vi "Main.vi"() -> ()   [LabVIEW 2018]
uses:
  Ddigit--enum.ctl
  Mmultiplier--enum.ctl
  Ttolerance--enum.ctl
  Number of Bands--number.ctl
  Ttemp Ccoeficient--enum.ctl
  In series--cluster.ctl
  Data--cluster.ctl
  E-Series Reader/Series Data--cluster.ctl
  Resistance Digits--cluster.ctl
  <vilib>/TABOADA/Event-Driven Queued SM/ED Queued State Machine/Queue State & Data (Array).vi
  <vilib>/Utility/error.llb/Error Cluster From Error Code.vi
  <vilib>/TABOADA/Event-Driven Queued SM/ED Queued State Machine/Queue State & Data (Single).vi
  <vilib>/ErrorRing/Error Ring.xnode
  Enum to Color Converters/Enum to Color Converters.lvlib
  E-Series Reader/E-Series Reader.lvlib
  Resistance Value/Resistance Value.lvlib
  Front Panel Interface/Front Panel Interface.lvlib
  <vilib>/TABOADA/Event-Driven Queued SM/ED Queued State Machine/ED Queued State Machine.lvlib
panel:
  out "RNV":dbl format="%#_6p"
  in  "Exit":bool
  out "T Rge":dbl caption="Tol Range [Ohm]" format="%_2p"
  out "Dev":dbl caption="Deviation [Ohm]" format="%_2p"
  out "UL":dbl caption="Upper Limit [Ohm]" format="%_3p"
  out "LL":dbl caption="Lower Limit [Ohm]" format="%_3p"
  out "Tol %":dbl caption="Tolerance (%)"
  out "In S":T1 caption="In Series"
  in  "Series Data File Name":string="e-series files names.ini"
  out "TC col":u32(colorbox) caption="TC"
  out "3D col":u32(colorbox) caption="3D"
  out "Tol col":u32(colorbox) caption="Tol"
  out "M col":u32(colorbox) caption="M"
  out "2D col":u32(colorbox) caption="2D"
  out "1D col":u32(colorbox) caption="1D"
  in  "Temp Coef":T2
  in  "3° Digit":T3
  in  "# Bands":T4=3 caption="Number of Bands" min=3 max=6 step=1
  out "N Val":dbl caption="Nominal [Ohm]" format="%#_3p"
  in  "Tolerance":T5=enum."Gold - 5%"
  in  "Multiplier":T6
  in  "2° Digit":T3
  in  "1° Digit":T3
  # "Resistor graphical representation"
  # "User Data Input"
  # "Calculated Resistor Specifications"
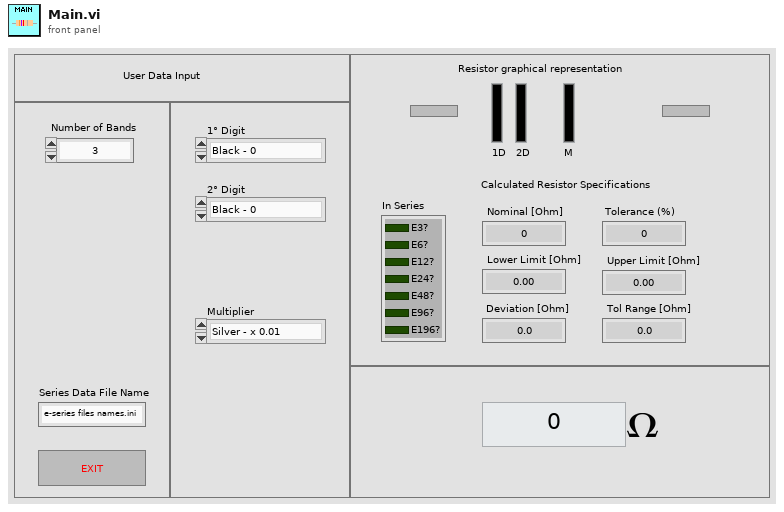
[diagram p1: front panel]
types:
  T1 = typedef "In series--cluster.ctl" = cluster{"E3?":bool, "E6?":bool, "E12?":bool, "E24?":bool, "E48?":bool, "E96?":bool, "E196?":bool}
  T2 = typedef "Ttemp Ccoeficient--enum.ctl" = enum16{"Grey - 1 ppm/K", "Violet - 5 ppm/K", "Blue - 10 ppm/K", "Green - 20 ppm/K", "Yellow - 25 ppm/K", "Orange - 15 ppm/K", "Red - 50 ppm/K", "Brown - 100 ppm/K", "Black - 250 ppm/K"}
  T3 = typedef "Ddigit--enum.ctl" = enum16{"Black - 0", "Brown - 1", "Red - 2", "Orange - 3", "Yellow - 4", "Green - 5", "Blue - 6", "Violet - 7", "Grey - 8", "White - 9"}
  T4 = typedef "Number of Bands--number.ctl" = u8
  T5 = typedef "Ttolerance--enum.ctl" = enum16{"Gray - 0.05%", "Violet - 0.1%", "Blue - 0.25%", "Green - 0.5%", "Brown - 1%", "Red - 2%", "Gold - 5%", "Silver - 10%", "None - 20%"}
  T6 = typedef "Mmultiplier--enum.ctl" = enum16{"Silver - x 0.01", "Gold - x 0.1 ", "Black - x 1", "Brown - x 10", "Red - x 100", "Orange - x 1k", "Yellow - x 10k", "Green - 100k", "Blue - x 1M", "Violet - x10 M", "Grey - x 100M", "White - x 1G"}
  T7 = typedef "Data--cluster.ctl" = cluster{"1D sel Refn":refnum<vi>, "2D sel Refn":refnum<vi>, "3D sel Refn":refnum<vi>, "M sel Refn":refnum<vi>, "Tol sel Refn":refnum<vi>, "TC sel Refn":refnum<vi>, "# Bands Refn":refnum<vi>, "1D col Refn":refnum<vi>, "2D col Refn":refnum<vi>, "3D col Refn":refnum<vi>, "M col Refn":refnum<vi>, "Tol col Refn":refnum<vi>, "TC col Refn":refnum<vi>, "# Bands":T4, "E-Series Data":T8, "In Series?":T1, "1D sel":T3, "2D sel":T3, "3D sel":T3, "M sel":T6, "Tol sel":T5, "TC sel":T2, "Tol %":dbl, "1D col":u32, "2D col":u32, "3D col":u32, "M col":u32, "Tol col":u32, "TC col":u32, "Nom Value":dbl, "Up Limit":dbl, "Lo Limit":dbl, "Deviation":dbl, "Tol Rge":dbl}
  T8 = typedef "E-Series Reader.lvlib/Series Data--cluster.ctl" = cluster{"E3":u16[], "E6":u16[], "E12":u16[], "E24":u16[], "E48":u16[], "E96":u16[], "E192":u16[]}
  T9 = typedef "Resistance Digits--cluster.ctl" = cluster{"LSD Digit":T3, "MID Digit":T3, "MSD Digit":T3}
  T10 = typedef "digit--enum.ctl" = enum16{"Black - 0", "Brown - 1", "Red - 2", "Orange - 3", "Yellow - 4", "Green - 5", "Blue - 6", "Violet - 7", "Grey - 8", "White - 9"}
  T11 = typedef "multiplier--enum.ctl" = enum16{"Silver - x 0.01", "Gold - x 0.1 ", "Black - x 1", "Brown - x 10", "Red - x 100", "Orange - x 1k", "Yellow - x 10k", "Green - 100k", "Blue - x 1M", "Violet - x10 M", "Grey - x 100M", "White - x 1G"}
  T12 = typedef "tolerance--enum.ctl" = enum16{"Gray - 0.05%", "Violet - 0.1%", "Blue - 0.25%", "Green - 0.5%", "Brown - 1%", "Red - 2%", "Gold - 5%", "Silver - 10%", "None - 20%"}
  T13 = typedef "temp coeficient--enum.ctl" = enum16{"Grey - 1 ppm/K", "Violet - 5 ppm/K", "Blue - 10 ppm/K", "Green - 20 ppm/K", "Yellow - 25 ppm/K", "Orange - 15 ppm/K", "Red - 50 ppm/K", "Brown - 100 ppm/K", "Black - 250 ppm/K"}
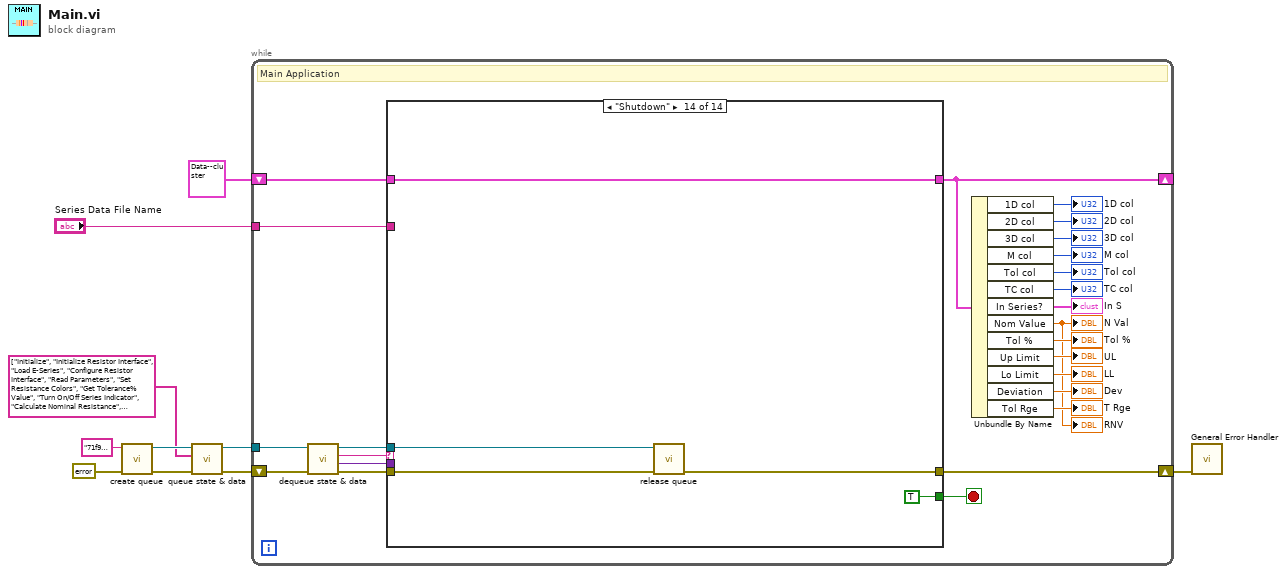
[diagram p0: block diagram]
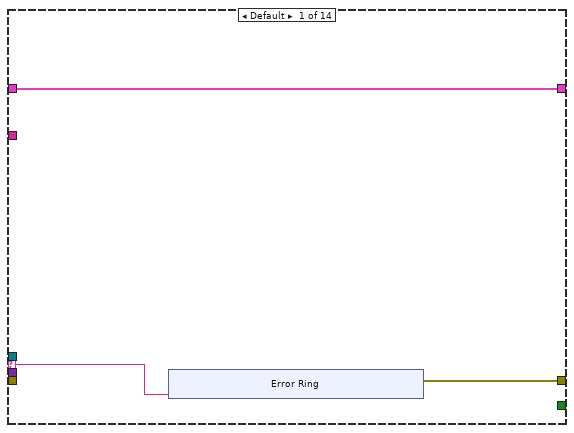
[diagram p2: hidden frame]
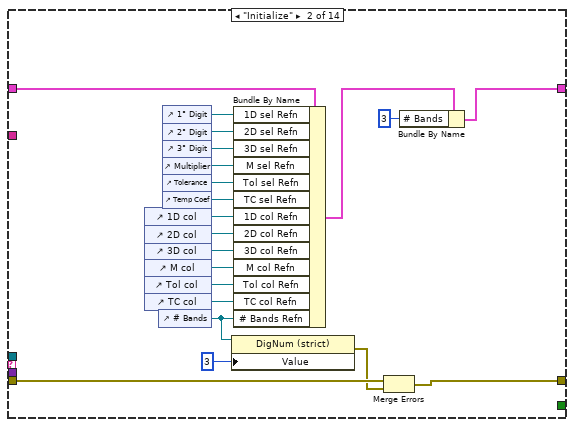
[diagram p3: hidden frame]
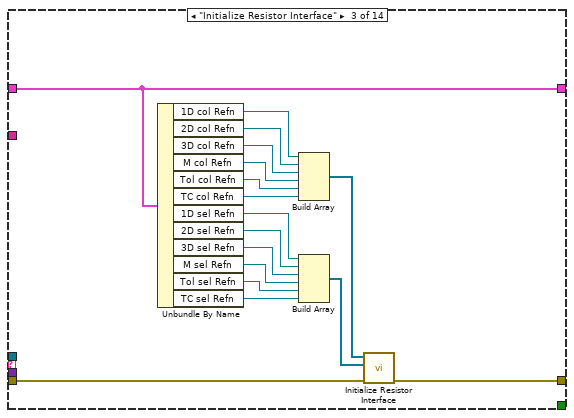
[diagram p4: hidden frame]
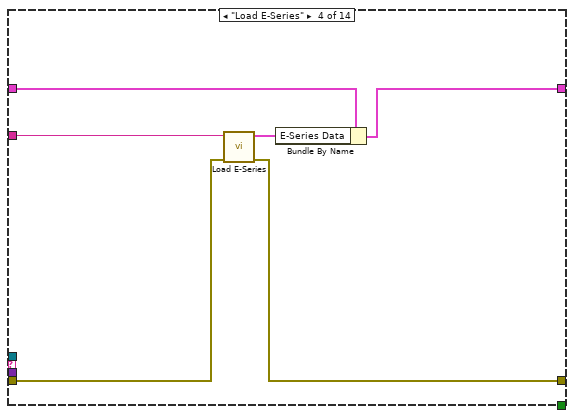
[diagram p5: hidden frame]
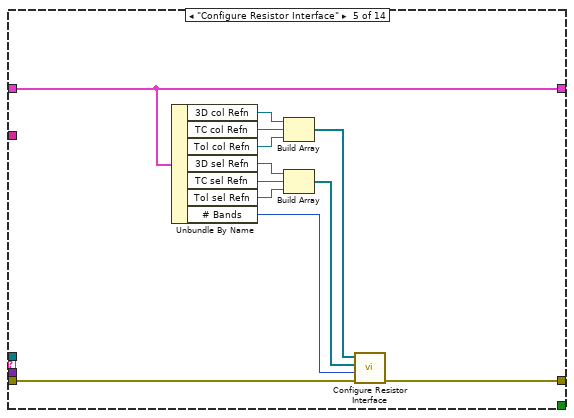
[diagram p6: hidden frame]
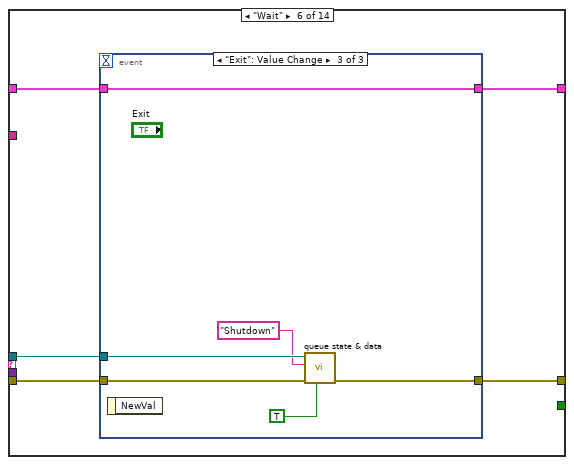
[diagram p7: hidden frame]
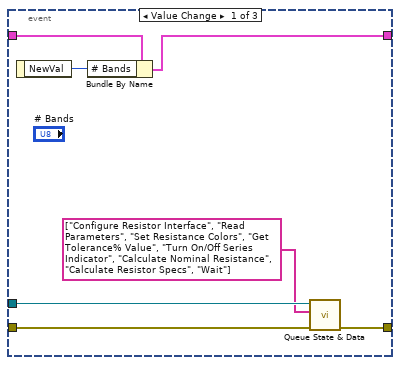
[diagram p8: hidden frame]
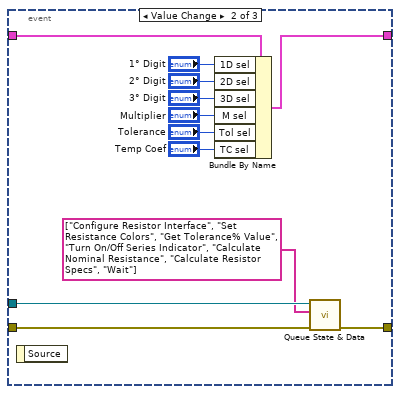
[diagram p9: hidden frame]
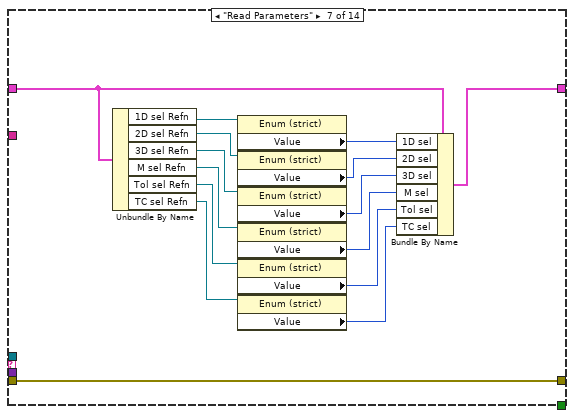
[diagram p10: hidden frame]
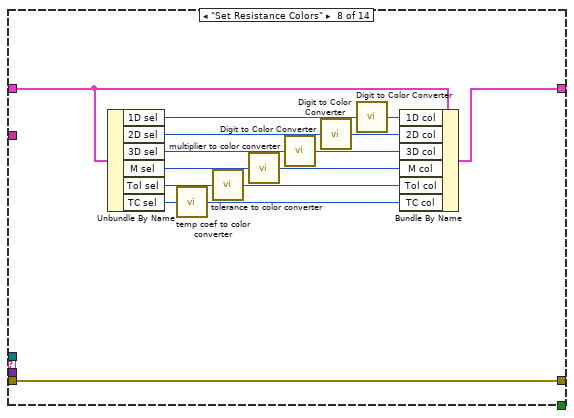
[diagram p11: hidden frame]
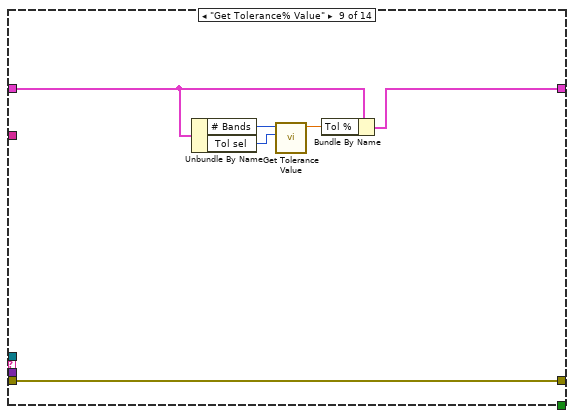
[diagram p12: hidden frame]
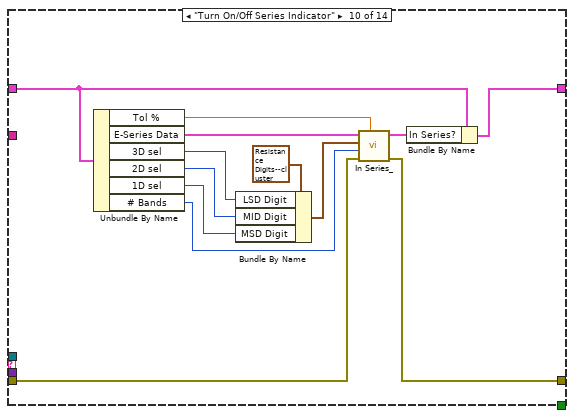
[diagram p13: hidden frame]
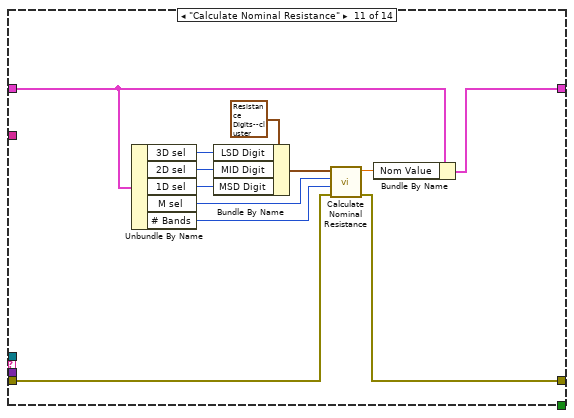
[diagram p14: hidden frame]
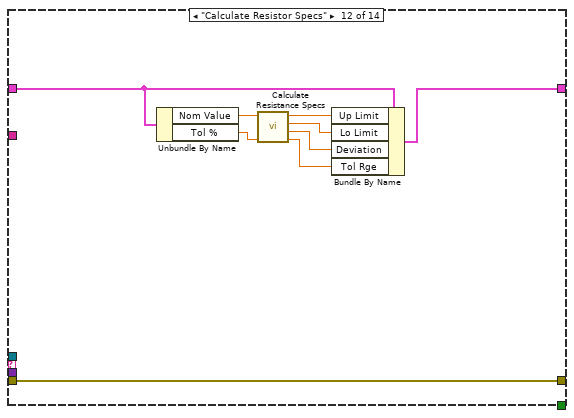
[diagram p15: hidden frame]
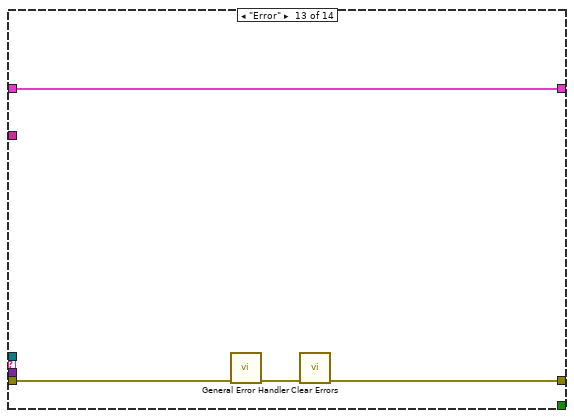
[diagram p16: hidden frame]
diagram:
  n1 = call <vilib>:"create queue.vi"("error in (no error)"=errorcluster {"status"=FALSE, "code"=0, "source"=""} ("error constant"), "name (unnamed)"="71f9ea68-780e-483a-a5bb-45874721e19e") -> ("error out"=w6:errorcluster, "queue out"=w4:refnum<queue>)  [unwired: 7 in, 1 out]
  n2 = call-poly <vilib>:"queue state & data.vi"("error in (no error)"=w6, "State Array"=string[] ["Initialize", "Initialize Resistor Interface", "Load E-Series", "Configure Resistor Interface", "Read Parameters", "Set Resistance Colors", "Get Tolerance% Value", "Turn On/Off Series Indicator", "Calculate Nominal Resistance", "Calculate Resistor Specs", "Wait"], "queue in"=w4) -> ("error out"=w7:errorcluster, "queue out"=w3:refnum<queue>)  [unwired: 7 in]
  n3 = while {
    shift-right: [w34] -> w9
    shift-left: w7 -> [w22]
    shift-right: [w24] -> _
    shift-left: T7 {"1D sel Refn"=refnum, "2D sel Refn"=refnum, "3D sel Refn"=refnum, "M sel Refn"=refnum, "Tol sel Refn"=refnum, "TC sel Refn"=refnum, "# Bands Refn"=refnum, "1D col Refn"=refnum, "2D col Refn"=refnum, "3D col Refn"=refnum, "M col Refn"=refnum, "Tol col Refn"=refnum, "TC col Refn"=refnum, "# Bands"=0, "E-Series Data"={"E3"=[], "E6"=[], "E12"=[], "E24"=[], "E48"=[], "E96"=[], "E192"=[]}, "In Series?"={"E3?"=FALSE, "E6?"=FALSE, "E12?"=FALSE, "E24?"=FALSE, "E48?"=FALSE, "E96?"=FALSE, "E196?"=FALSE}, "1D sel"=enum."Black - 0", "2D sel"=enum."Black - 0", "3D sel"=enum."Black - 0", "M sel"=enum."Silver - x 0.01", "Tol sel"=enum."Gray - 0.05%", "TC sel"=enum."Grey - 1 ppm/K", "Tol %"=0.0, "1D col"=0, "2D col"=0, "3D col"=0, "M col"=0, "Tol col"=0, "TC col"=0, "Nom Value"=0.0, "Up Limit"=0.0, "Lo Limit"=0.0, "Deviation"=0.0, "Tol Rge"=0.0} -> [w25]
    tunnel: "Series Data File Name" -> [w26]
    tunnel: w3 -> [w23]
    stop <- w33 stop-if-true
    # "Main Application"
    n4 = call <vilib>:"dequeue state & data.vi"("error in (no error)"=w22, "queue in"=w23) -> ("error out"=w20:errorcluster, "State Data"=w18:variant, "State"=w19:string, "queue out"=w21:refnum<queue>)  [unwired: 6 in]
    n5 = case shown="\"Shutdown\"" w19 {
      selector: w19 -> [w36 _ _ _ _ _ _ _ _ _ _ _ _ _]
      tunnel: w20 -> [_ w65 w76 w84 w95 w103 w145 w159 w166 w169 w182 w200 w202 w207]
      tunnel: [w35 w49 w75 w86 w96 w102 w145 w159 w166 w168 w181 w200 w203 w206] -> w34
      tunnel: w25 -> [w37 w64 w82 w88 w100 w105 w143 w157 w165 w172 w191 w199 w204 w209]
      tunnel: [w37 w46 w82 w87 w100 w104 w144 w156 w163 w170 w190 w198 w204 w209] -> w24
      tunnel: [_ _ _ _ _ _ _ _ _ _ _ _ _ TRUE] -> w33
      tunnel: w26 -> [_ _ _ w83 _ _ _ _ _ _ _ _ _ _]
      tunnel: w21 -> [_ _ _ _ _ w101 _ _ _ _ _ _ _ w205]
      tunnel: w18 -> [_ _ _ _ _ _ _ _ _ _ _ _ _ _]
      frame Default {
        n6 = xnode ("Error Ring")("parameter 0"=w36) -> ("error out"=w35:errorcluster)
      }
      frame "Initialize" {
        n7 = control-ref of="1D col"() -> (w60:refnum<vi>)
        n8 = control-ref of="2D col"() -> (w59:refnum<vi>)
        n9 = control-ref of="3D col"() -> (w58:refnum<vi>)
        n10 = control-ref of="M col"() -> (w57:refnum<vi>)
        n11 = control-ref of="Tol col"() -> (w56:refnum<vi>)
        n12 = control-ref of="TC col"() -> (w55:refnum<vi>)
        n13 = control-ref of="# Bands"() -> (w51:refnum<vi>)
        n14 = control-ref of="1° Digit"() -> (w52:refnum<vi>)
        n15 = control-ref of="2° Digit"() -> (w53:refnum<vi>)
        n16 = control-ref of="3° Digit"() -> (w54:refnum<vi>)
        n17 = control-ref of="Multiplier"() -> (w63:refnum<vi>)
        n18 = control-ref of="Tolerance"() -> (w62:refnum<vi>)
        n19 = control-ref of="Temp Coef"() -> (w61:refnum<vi>)
        n20 = property class="DigNum (strict)"(reference=w51, "Value"=T4 3 ("Number of Bands")) -> (error out=w48:errorcluster)  [unwired: 1 in, 1 out]
        n21 = Bundle By Name(cluster=w64, "1D sel Refn"=w52, "2D sel Refn"=w53, "3D sel Refn"=w54, "M sel Refn"=w63, "Tol sel Refn"=w62, "TC sel Refn"=w61, "1D col Refn"=w60, "2D col Refn"=w59, "3D col Refn"=w58, "M col Refn"=w57, "Tol col Refn"=w56, "TC col Refn"=w55, "# Bands Refn"=w51) -> (w47:T7)
        n22 = Merge Errors(w65, w48) -> (w49:errorcluster)
        n23 = Bundle By Name(cluster=w47, "# Bands"=T4 3) -> (w46:T7)
      }
      frame "Initialize Resistor Interface" {
        n24 = Unbundle By Name(w82) -> ("1D col Refn"=w81:refnum<vi>, "2D col Refn"=w80:refnum<vi>, "3D col Refn"=w79:refnum<vi>, "M col Refn"=w73:refnum<vi>, "Tol col Refn"=w74:refnum<vi>, "TC col Refn"=w78:refnum<vi>, "1D sel Refn"=w72:refnum<vi>, "2D sel Refn"=w71:refnum<vi>, "3D sel Refn"=w70:refnum<vi>, "M sel Refn"=w69:refnum<vi>, "Tol sel Refn"=w68:refnum<vi>, "TC sel Refn"=w67:refnum<vi>)
        n25 = Build Array(w81, w80, w79, w73, w74, w78) -> (w77:refnum<vi>[])
        n26 = Build Array(w72, w71, w70, w69, w68, w67) -> (w66:refnum<vi>[])
        n27 = call "Initialize Resistor Interface.vi"("error in (no error)"=w76, "Enum Refnum"=w66, "Color Box Refnum"=w77) -> ("error out"=w75:errorcluster)  [unwired: 8 in]
      }
      frame "Load E-Series" {
        n28 = call "Load E-Series.vi"("error in (no error)"=w84, "INI File"=w83) -> ("error out"=w86:errorcluster, "E-Series Data"=w85:T8)  [unwired: 8 in]
        n29 = Bundle By Name(cluster=w88, "E-Series Data"=w85) -> (w87:T7)
      }
      frame "Configure Resistor Interface" {
        n30 = Unbundle By Name(w100) -> ("3D col Refn"=w98:refnum<vi>, "TC col Refn"=w99:refnum<vi>, "Tol col Refn"=w97:refnum<vi>, "3D sel Refn"=w92:refnum<vi>, "TC sel Refn"=w93:refnum<vi>, "Tol sel Refn"=w91:refnum<vi>, "# Bands"=w89:T4)
        n31 = Build Array(w98, w99, w97) -> (w94:refnum<vi>[])
        n32 = Build Array(w92, w93, w91) -> (w90:refnum<vi>[])
        n33 = call "Configure Resistor Interface.vi"("error in (no error)"=w95, "Number of Bands in"=w89, "Enum Refnum"=w90, "Color Box Refnum"=w94) -> ("error out"=w96:errorcluster)  [unwired: 7 in]
      }
      frame "Wait" {
        n34 = event shown="[2] \"Exit\": Value Change" {
          selector: _ -> [_ _ _]
          dyn-events: _ -> [_ _ _]
          timeout: _ -> [_ _ _]
          tunnel: w105 -> [w112 w124 w130]
          tunnel: [w111 w123 w130] -> w104
          tunnel: w103 -> [w109 w116 w128]
          tunnel: [w108 w115 w127] -> w102
          tunnel: w101 -> [w107 w114 w129]
          event Value Change {
            n35 = event-data() -> ("NewVal"=w110:T4)  [unwired: 1 in]
            n36 = Bundle By Name(cluster=w112, "# Bands"=w110) -> (w111:T7)
            n37 = call-poly <vilib>:"Queue State & Data.vi"("error in (no error)"=w109, "State Array"=string[] ["Configure Resistor Interface", "Read Parameters", "Set Resistance Colors", "Get Tolerance% Value", "Turn On/Off Series Indicator", "Calculate Nominal Resistance", "Calculate Resistor Specs", "Wait"], "queue in"=w107) -> ("error out"=w108:errorcluster)  [unwired: 7 in, 1 out]
          }
          event Value Change {
            n38 = event-data() -> ()  [unwired: 1 in, 1 out]
            n39 = Bundle By Name(cluster=w124, "1D sel"="1° Digit", "2D sel"="2° Digit", "3D sel"="3° Digit", "M sel"="Multiplier", "Tol sel"="Tolerance", "TC sel"="Temp Coef") -> (w123:T7)
            n40 = call-poly <vilib>:"Queue State & Data.vi"("error in (no error)"=w116, "State Array"=string[] ["Configure Resistor Interface", "Set Resistance Colors", "Get Tolerance% Value", "Turn On/Off Series Indicator", "Calculate Nominal Resistance", "Calculate Resistor Specs", "Wait"], "queue in"=w114) -> ("error out"=w115:errorcluster)  [unwired: 7 in, 1 out]
          }
          event "Exit": Value Change {
            n41 = event-data() -> ()  [unwired: 1 in, 1 out]
            n42 = call-poly <vilib>:"queue state & data.vi"("Priority State? (F)"=TRUE, "error in (no error)"=w128, "State"="Shutdown", "queue in"=w129) -> ("error out"=w127:errorcluster)  [unwired: 6 in, 1 out]
          }
        }
      }
      frame "Read Parameters" {
        n43 = Unbundle By Name(w143) -> ("1D sel Refn"=w142:refnum<vi>, "2D sel Refn"=w140:refnum<vi>, "3D sel Refn"=w139:refnum<vi>, "M sel Refn"=w136:refnum<vi>, "Tol sel Refn"=w135:refnum<vi>, "TC sel Refn"=w134:refnum<vi>)
        n44 = property class="Enum (strict)"(reference=w142) -> ("Value"=w141:T10)  [unwired: 1 in, 2 out]
        n45 = property class="Enum (strict)"(reference=w140) -> ("Value"=w138:T10)  [unwired: 1 in, 2 out]
        n46 = property class="Enum (strict)"(reference=w139) -> ("Value"=w137:T10)  [unwired: 1 in, 2 out]
        n47 = property class="Enum (strict)"(reference=w136) -> ("Value"=w133:T11)  [unwired: 1 in, 2 out]
        n48 = property class="Enum (strict)"(reference=w135) -> ("Value"=w132:T12)  [unwired: 1 in, 2 out]
        n49 = property class="Enum (strict)"(reference=w134) -> ("Value"=w131:T13)  [unwired: 1 in, 2 out]
        n50 = Bundle By Name(cluster=w143, "1D sel"=w141, "2D sel"=w138, "3D sel"=w137, "M sel"=w133, "Tol sel"=w132, "TC sel"=w131) -> (w144:T7)
      }
      frame "Set Resistance Colors" {
        n51 = Unbundle By Name(w157) -> ("1D sel"=w160:T3, "2D sel"=w158:T3, "3D sel"=w149:T3, "M sel"=w153:T6, "Tol sel"=w152:T5, "TC sel"=w147:T2)
        n52 = call "temp coef to color converter.vi"("TC select"=w147) -> ("TC Color"=w146:u32)  [unwired: 6 in]
        n53 = call "tolerance to color converter.vi"("To select"=w152) -> ("Tol Color"=w151:u32)  [unwired: 6 in]
        n54 = call "multiplier to color converter.vi"("Mul select"=w153) -> ("Mult Color"=w150:u32)  [unwired: 6 in]
        n55 = call "Digit to Color Converter.vi"("D select"=w149) -> ("D Color"=w148:u32)  [unwired: 4 in]
        n56 = call "Digit to Color Converter.vi"("D select"=w158) -> ("D Color"=w154:u32)  [unwired: 4 in]
        n57 = call "Digit to Color Converter.vi"("D select"=w160) -> ("D Color"=w155:u32)  [unwired: 4 in]
        n58 = Bundle By Name(cluster=w157, "1D col"=w155, "2D col"=w154, "3D col"=w148, "M col"=w150, "Tol col"=w151, "TC col"=w146) -> (w156:T7)
      }
      frame "Get Tolerance% Value" {
        n59 = Unbundle By Name(w165) -> ("# Bands"=w162:T4, "Tol sel"=w161:T5)
        n60 = call "Get Tolerance Value.vi"("Tol sel"=w161, "# Bands"=w162) -> ("Numeric"=w164:dbl)  [unwired: 9 in]
        n61 = Bundle By Name(cluster=w165, "Tol %"=w164) -> (w163:T7)
      }
      frame "Turn On/Off Series Indicator" {
        n62 = Unbundle By Name(w172) -> ("Tol %"=w167:dbl, "E-Series Data"=w179:T8, "3D sel"=w177:T3, "2D sel"=w176:T3, "1D sel"=w175:T3, "# Bands"=w173:T4)
        n63 = Bundle By Name(cluster=T9 {"LSD Digit"=enum."Black - 0", "MID Digit"=enum."Black - 0", "MSD Digit"=enum."Black - 0"} ("Resistance Digits"), "LSD Digit"=w177, "MID Digit"=w176, "MSD Digit"=w175) -> (w174:T9)
        n64 = call "In Series_.vi"("Tolerance (%)"=w167, "error in (no error)"=w169, "Number of Bands"=w173, "Resistance Digits"=w174, "E-Series Data"=w179) -> ("error out"=w168:errorcluster, "In Series?"=w171:T1)  [unwired: 5 in]
        n65 = Bundle By Name(cluster=w172, "In Series?"=w171) -> (w170:T7)
      }
      frame "Calculate Nominal Resistance" {
        n66 = Unbundle By Name(w191) -> ("3D sel"=w183:T3, "2D sel"=w186:T3, "1D sel"=w185:T3, "M sel"=w188:T6, "# Bands"=w180:T4)
        n67 = Bundle By Name(cluster=T9 {"LSD Digit"=enum."Black - 0", "MID Digit"=enum."Black - 0", "MSD Digit"=enum."Black - 0"} ("Resistance Digits"), "LSD Digit"=w183, "MID Digit"=w186, "MSD Digit"=w185) -> (w184:T9)
        n68 = call "Calculate Nominal Resistance.vi"("error in (no error)"=w182, "Number of Bands"=w180, "M sel"=w188, "Resistance Digits"=w184) -> ("error out"=w181:errorcluster, "Nominal Value"=w189:dbl)  [unwired: 6 in]
        n69 = Bundle By Name(cluster=w191, "Nom Value"=w189) -> (w190:T7)
      }
      frame "Calculate Resistor Specs" {
        n70 = Unbundle By Name(w199) -> ("Nom Value"=w196:dbl, "Tol %"=w193:dbl)
        n71 = call "Calculate Resistance Specs.vi"("Tol %"=w193, "Nom Value"=w196) -> ("Tol Range"=w192:dbl, "Deviation"=w197:dbl, "Lower Limit"=w194:dbl, "Upper Limit"=w195:dbl)  [unwired: 6 in]
        n72 = Bundle By Name(cluster=w199, "Up Limit"=w195, "Lo Limit"=w194, "Deviation"=w197, "Tol Rge"=w192) -> (w198:T7)
      }
      frame "Error" {
        n73 = call <vilib>:"General Error Handler.vi"("error in (no error)"=w202) -> ("error out"=w201:errorcluster)  [unwired: 10 in, 4 out]
        n74 = call <vilib>:"Clear Errors.vi"("error in (no error)"=w201) -> ("error out"=w203:errorcluster)  [unwired: 5 in, 1 out]
      }
      frame "Shutdown" {
        n75 = call <vilib>:"release queue.vi"("error in (no error)"=w207, "queue in"=w205) -> ("error out"=w206:errorcluster)  [unwired: 9 in]
      }
    }
    n76 = Unbundle By Name(w24) -> ("1D col"=→"1D col":u32, "2D col"=→"2D col":u32, "3D col"=→"3D col":u32, "M col"=→"M col":u32, "Tol col"=→"Tol col":u32, "TC col"=→"TC col":u32, "In Series?"=→"In S":T1, "Nom Value"=→"N Val" →"RNV":dbl, "Tol %"=→"Tol %":dbl, "Up Limit"=→"UL":dbl, "Lo Limit"=→"LL":dbl, "Deviation"=→"Dev":dbl, "Tol Rge"=→"T Rge":dbl)
  }
  n77 = call <vilib>:"General Error Handler.vi"("error in (no error)"=w9) -> ()  [unwired: 10 in, 5 out]
